vi "StopSessionImmediately.vi"(11 "Session in":refnum<class "Session.lvclass">) -> (0 "error out":errorcluster, 3 "Session out":refnum<class "Session.lvclass">)   [LabVIEW 2013, in "MQTT Server.lvlib" / "Session.lvclass"]
uses:
  Session.lvclass
  Session.lvclass/Session.ctl
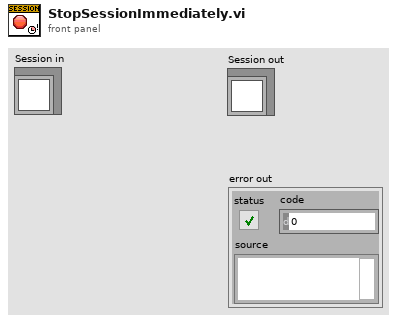
[diagram p1: front panel]
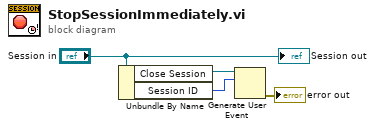
[diagram p0: block diagram]
diagram:
  n1 = Unbundle By Name("Session in") -> ("Close Session"=w3:refnum<user-event>, "Session ID"=w4:i32)
  n2 = Generate User Event(user event=w3, event data cluster=w4) -> (error out=→"error out":errorcluster)  [unwired: 2 in, 1 out]
  "Session out" <- "Session in"
